vi "PC.vi"() -> ()   [LabVIEW 2016]
doc: "Demonstrates how to use User Datagram Protocol (UDP) to send data to the myRIO target."
panel:
  out "datos enviados":bool[](array[boolean])
  in  "Stop Button":bool
  out "motores":string
  out "error out":errorcluster
  # "Overview: Demonstrates how to use User Datagram Protocol (UDP) to send data to the myRIO target.\nInstructions:\n1. Verify the value of Target IP Address. If it is incorrect, specify the correct value.\n2. (Optional) To broadcast data to several myRIO targets without specifying their IP addresses, set the value of Target IP Address to one of the following values:\n    - 255.255.255.255\n    - 192.168.1.255, if your IP address is in the form 192.168.1.x.\n3. Run the VI.\n4. Open RT Main.vi and follow its front panel instructions.\n5. Click Stop to stop the VI."
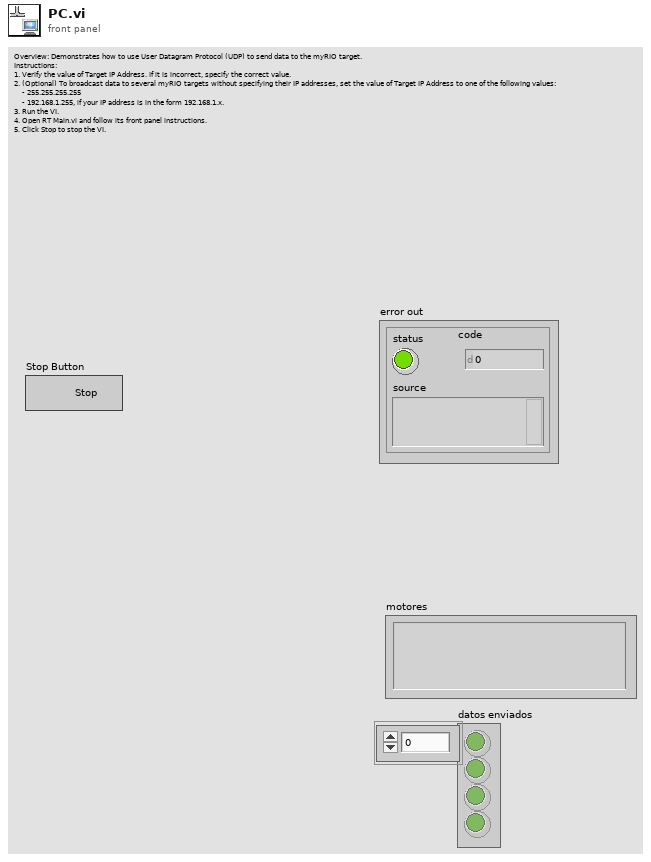
[diagram p1: front panel]
types:
  T1 = enum16{"Read", "Write", "ReadWrite", "BufferedRead", "BufferedReadWrite"}
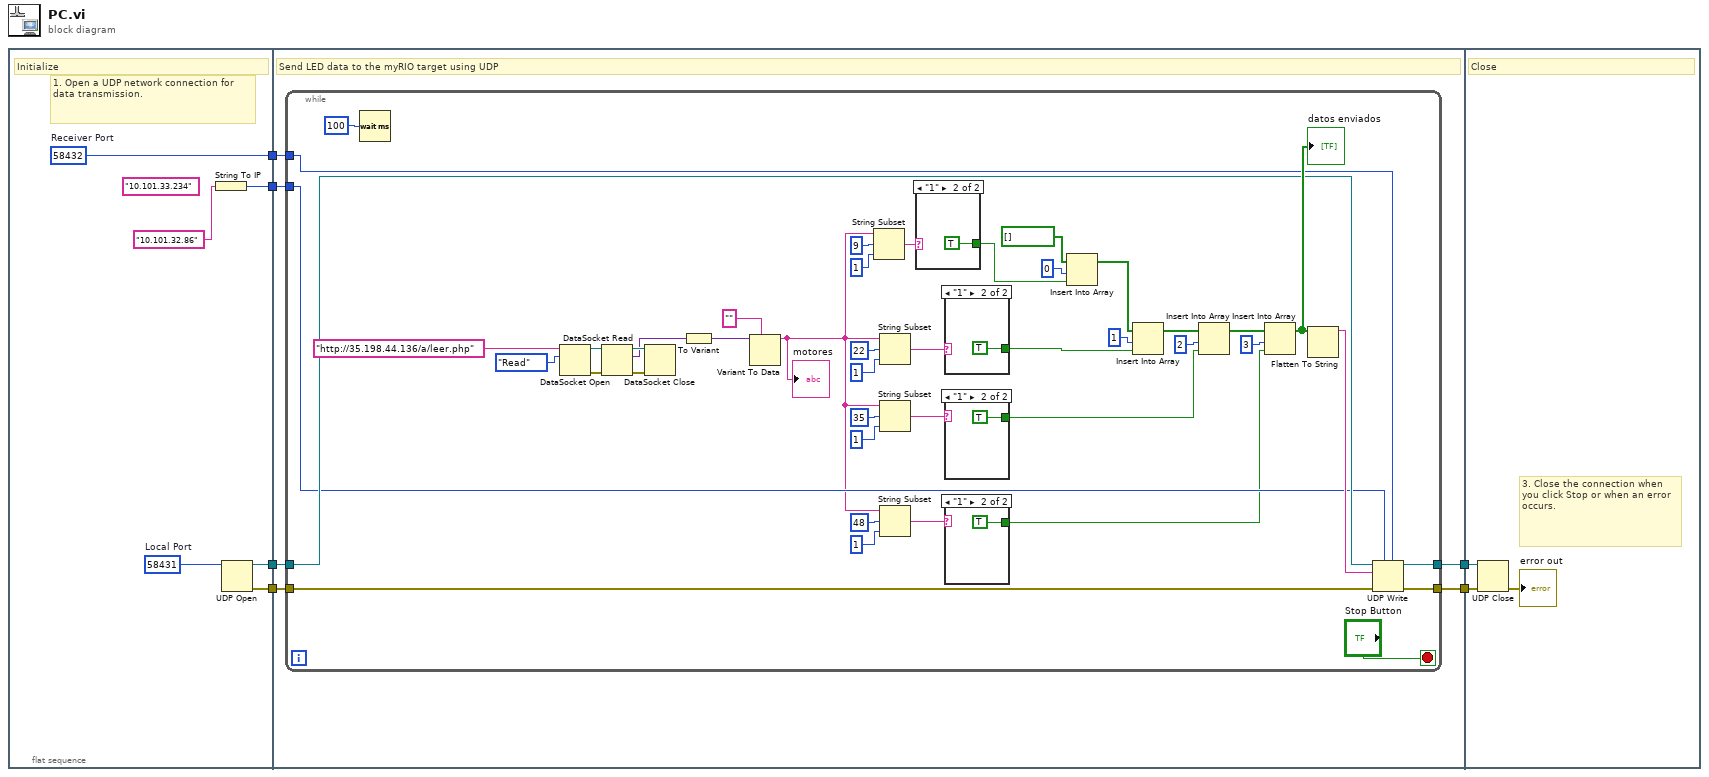
[diagram p0: block diagram]
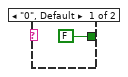
[diagram p2: hidden frame]
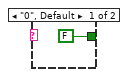
[diagram p3: hidden frame]
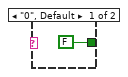
[diagram p4: hidden frame]
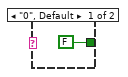
[diagram p5: hidden frame]
diagram:
  n1 = flat-sequence {
    tunnel: [w12] -> w4
    tunnel: [w11] -> w3
    tunnel: [w9] -> w2
    tunnel: [w8] -> w1
    tunnel: [w13] -> w6
    tunnel: [w14] -> w5
    tunnel: w4 -> [w17]
    tunnel: w3 -> [w18]
    tunnel: w2 -> [w16]
    tunnel: w1 -> [w15]
    tunnel: w6 -> [w72]
    tunnel: w5 -> [w73]
    frame #0 {
      (unwired) "10.101.33.234"
      w8 = u16 58432  # Receiver Port
      w10 = u16 58431  # Local Port
      # "1. Open a UDP network connection for data transmission."
      # "Initialize"
      n2 = String To IP(1:"10.101.32.86") -> (0:w9:u32)
      n3 = UDP Open(11:w10) -> (port=w12:refnum<k16>, 0:w11:errorcluster)  [unwired: 4 in, 1 out]
    }
    frame #1 {
      # "Send LED data to the myRIO target using UDP"
      n4 = while {
        tunnel: w18 -> [w29]
        tunnel: w17 -> [w28]
        tunnel: w16 -> [w27]
        tunnel: w15 -> [w26]
        tunnel: [w25] -> w14
        tunnel: [w24] -> w13
        stop <- "Stop Button" stop-if-true
        n5 = Wait (ms)(milliseconds to wait=u32 100) -> ()  [unwired: 1 out]
        n6 = DataSocket Open(10:T1."Read" ("mode"), 11:"http://35.198.44.136/a/leer.php" ("URL")) -> (0:w59:errorcluster, 3:w60:refnum<k13>)  [unwired: 2 in]
        n7 = DataSocket Read(8:w59, 11:w60) -> (0:w61:errorcluster, 2:w58:variant, 3:w62:refnum<k13>)  [unwired: 3 in, 4 out]
        n8 = DataSocket Close(8:w61, 11:w62) -> ()  [unwired: 1 in, 2 out]
        n9 = To Variant(anything=w58) -> (Variant=w57:variant)
        n10 = Variant To Data(type="", Variant=w57) -> (data=w23:string)  [unwired: 1 in, 1 out]
        "motores" <- w23
        n11 = String Subset(string=w23, offset (0)=9, length (rest)=1 ("length (rest)")) -> (substring=w37:string)
        n12 = String Subset(string=w23, offset (0)=22, length (rest)=1 ("length (rest)")) -> (substring=w36:string)
        n13 = String Subset(string=w23, offset (0)=35, length (rest)=1 ("length (rest)")) -> (substring=w35:string)
        n14 = String Subset(string=w23, offset (0)=48, length (rest)=1 ("length (rest)")) -> (substring=w22:string)
        n15 = case shown="\"1\"" w37 {
          tunnel: [FALSE TRUE] -> w34
          frame "0", Default {
          }
          frame "1" {
          }
        }
        n16 = case shown="\"1\"" w36 {
          tunnel: [FALSE TRUE] -> w33
          frame "0", Default {
          }
          frame "1" {
          }
        }
        n17 = case shown="\"1\"" w35 {
          tunnel: [FALSE TRUE] -> w32
          frame "0", Default {
          }
          frame "1" {
          }
        }
        n18 = case shown="\"1\"" w22 {
          tunnel: [FALSE TRUE] -> w19
          frame "0", Default {
          }
          frame "1" {
          }
        }
        n19 = Insert Into Array(array=bool[] [], index=0, new element=w34) -> (w41:bool[])
        n20 = Insert Into Array(array=w41, index=1, new element=w33) -> (w40:bool[])
        n21 = Insert Into Array(array=w40, index=2, new element=w32) -> (w39:bool[])
        n22 = Insert Into Array(array=w39, index=3, new element=w19) -> (w31:bool[])
        "datos enviados" <- w31
        n23 = Flatten To String(anything=w31) -> (data string=w30:string)  [unwired: 3 in, 2 out]
        n24 = UDP Write(address=w27, port or service name=w26, connection ID=w28, data in=w30, 8:w29) -> (error out=w24:errorcluster, 3:w25:refnum<k16>)  [unwired: 1 in]
      }
    }
    frame #2 {
      # "3. Close the connection when you click Stop or when an error occurs."
      # "Close"
      n25 = UDP Close(connection ID=w73, 8:w72) -> (error out=→"error out":errorcluster)  [unwired: 1 out]
    }
  }
